vi "Create NT Enum.vi"(8 "error in":errorcluster) -> (0 "error out":errorcluster, 3 "PV Data out":refnum<class "PV Data.lvclass">)   [LabVIEW 2020, in "PV Access.lvlib" / "PV Data.lvlib" / "PV Data.lvclass"]
uses:
  PV Data.lvclass
  PV Data.lvclass/PV Data.ctl
  PV Access.lvlib
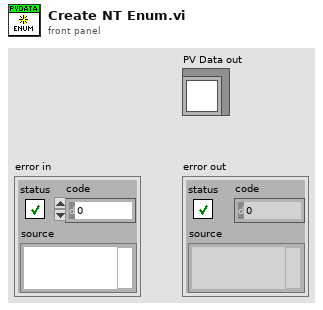
[diagram p1: front panel]
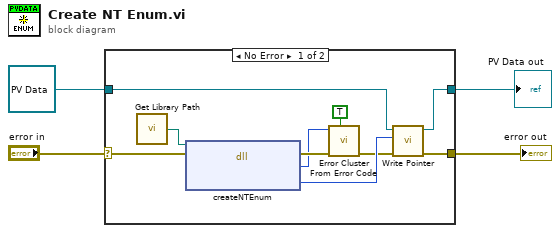
[diagram p0: block diagram]
diagram:
  n1 = case shown="No Error" "error in" {
    selector: "error in" -> [w14 w16]
    tunnel: [w6 w16] -> w4
    tunnel: refnum<class "PV Data.lvclass"> refnum ("PV Data in") -> [w8 w15]
    tunnel: [w7 w15] -> w1
    frame No Error {
      n2 = call "Get Library Path.vi"() -> ("Path"=w10:path)  [unwired: 1 in]
      n3 = dll-call lib="?" fn="createNTEnum" ("createNT Scalar")(path in=w10, error in=w14) -> (error out=w12:errorcluster, "err_code"=w11:i32, "value"=w9:i64)  [unwired: 2 in, 1 out]
      n4 = call <vilib>:"Error Cluster From Error Code.vi"("show call chain? (False)"=TRUE, "error in (no error)"=w12, "error code (0)"=w11) -> ("error out"=w5:errorcluster)  [unwired: 6 in]
      n5 = call-dynamic "Write Pointer.vi"("error in (no error)"=w5, "Pointer"=w9, "Pointer Base in"=w8) -> ("error out"=w6:errorcluster, "Pointer Base out"=w7:refnum<class "PV Data.lvclass">)  [unwired: 7 in]
    }
    frame Error {
    }
  }
  "error out" <- w4
  "PV Data out" <- w1
